vi "Initialize HW.vi"(8 "error in (no error)":errorcluster, 11 "Actuator in":refnum<class "Actuator.lvclass">) -> (0 "error out":errorcluster, 3 "Actuator out":refnum<class "Actuator.lvclass">)   [LabVIEW 2020, in "Actuator.lvclass"]
uses:
  Actuator.lvclass
  General Hardware.lvclass
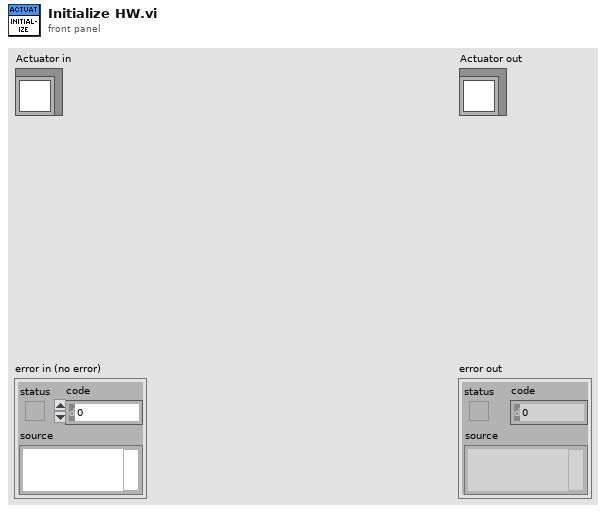
[diagram p1: front panel]
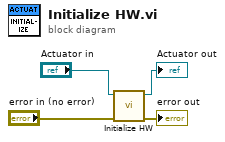
[diagram p0: block diagram]
diagram:
  n1 = call-parent "Initialize HW.vi"("error in (no error)"="error in (no error)", "General Hardware in"="Actuator in") -> ("error out"=→"error out":errorcluster, "General Hardware out"=→"Actuator out":refnum<class "Actuator.lvclass">)  [unwired: 8 in]
